vi "Status.TEST - Simple Text Status Indicator.vi"() -> ()   [LabVIEW 2024, in "EQMF.lvlib" / "Status Utils.lvlib"]
uses:
  Status Utils.lvlib
panel:
  in  "Event":enum16{"None", "Warning", "Error"}(ring)
  out "Status error out":errorcluster
  out "Inst error out":errorcluster
  out "InsX Status":string caption="InstrumentX"
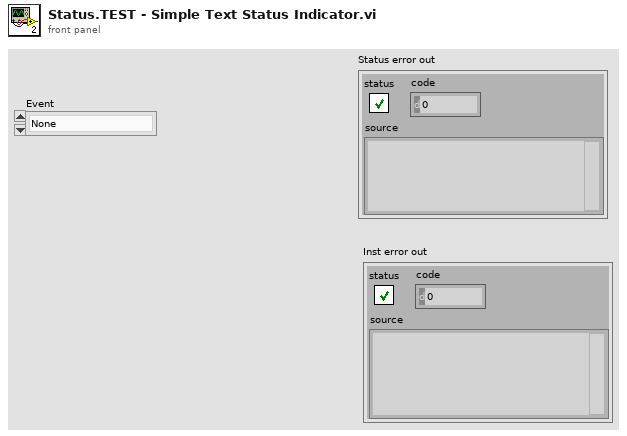
[diagram p1: front panel]
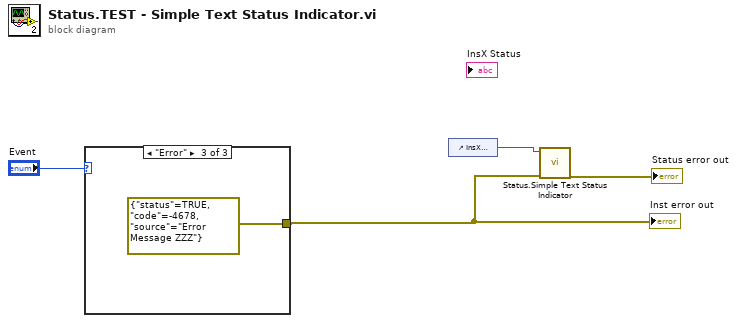
[diagram p0: block diagram]
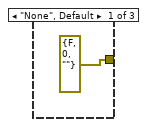
[diagram p2: hidden frame]
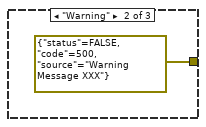
[diagram p3: hidden frame]
diagram:
  n1 = case shown="\"Error\"" "Event" {
    tunnel: [errorcluster {"status"=FALSE, "code"=0, "source"=""} ("error constant") errorcluster {"status"=FALSE, "code"=500, "source"="Warning Message XXX"} ("error constant") errorcluster {"status"=TRUE, "code"=-4678, "source"="Error Message ZZZ"} ("error constant")] -> w1
    frame "None", Default {
    }
    frame "Warning" {
    }
    frame "Error" {
    }
  }
  "Inst error out" <- w1
  n2 = control-ref of="InsX Status"() -> (w4:refnum<vi>)
  n3 = call "Status.Simple Text Status Indicator.vi"("error in"=w1, "Status TextBox"=w4) -> ("error out"=→"Status error out":errorcluster)  [unwired: 9 in]
